vi "Afficheur.vi"() -> ()   [LabVIEW 2013]
uses:
  <vilib>/DAQmx/read.llb/DAQmx Read (Analog Wfm 1Chan NSamp).vi
  <vilib>/DAQmx/create/channels.llb/DAQmx Create Channel (AI-Voltage-Basic).vi
  <vilib>/DAQmx/configure/timing.llb/DAQmx Timing (Sample Clock).vi
  <vilib>/measure/matone.llb/Extract Single Tone Information 1 Chan.vi
  <vilib>/DAQmx/miscellaneous.llb/DAQmx Fill In Error Info.vi
  <vilib>/express/express analysis/Spectral/Block/exnSpectralBlock spectral measurements PSD poly.vi
  <vilib>/express/express analysis/Spectral/Block/exnSpectralBlock spectral measurements PSD WFM.vi
  <vilib>/express/express analysis/Spectral/XNode/ExpressSpectralMeasurementsBlockNode.xnode
  <vilib>/measure/NI_MAPro.lvlib
panel:
  in  "fenetre":dbl
  out "indice fractionnaire ou x":dbl
  out "Y":dbl[](array[numeric])
  out "Final Waveform":waveform(dbl)(graph)
  out "Valeur efficace":dbl
  out "?":cluster{"f0":dbl, "df":dbl, "magnitude":dbl[]}(graph)
  out "mean":dbl caption="moyenne" format="%0.2f"
  out "Fréquence":dbl
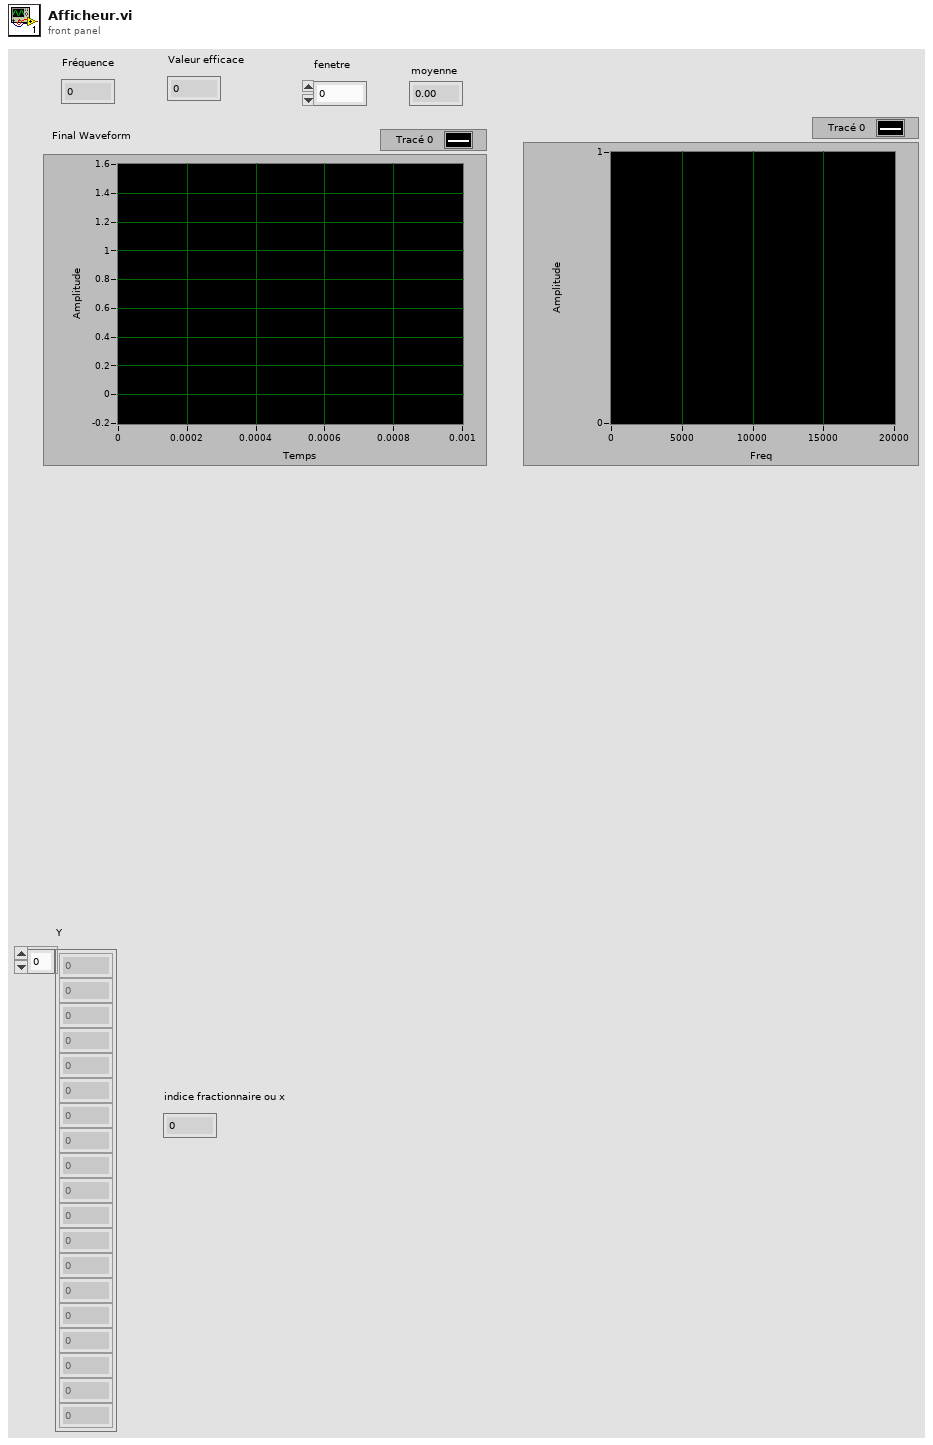
[diagram p1: front panel]
types:
  T1 = cluster{"averaging mode":u16, "weighting mode":u16, "number of averages":u32}
  T2 = cluster{"dB On (F)":bool, "unwrap phase (F)":bool, "convert to degree (F)":bool}
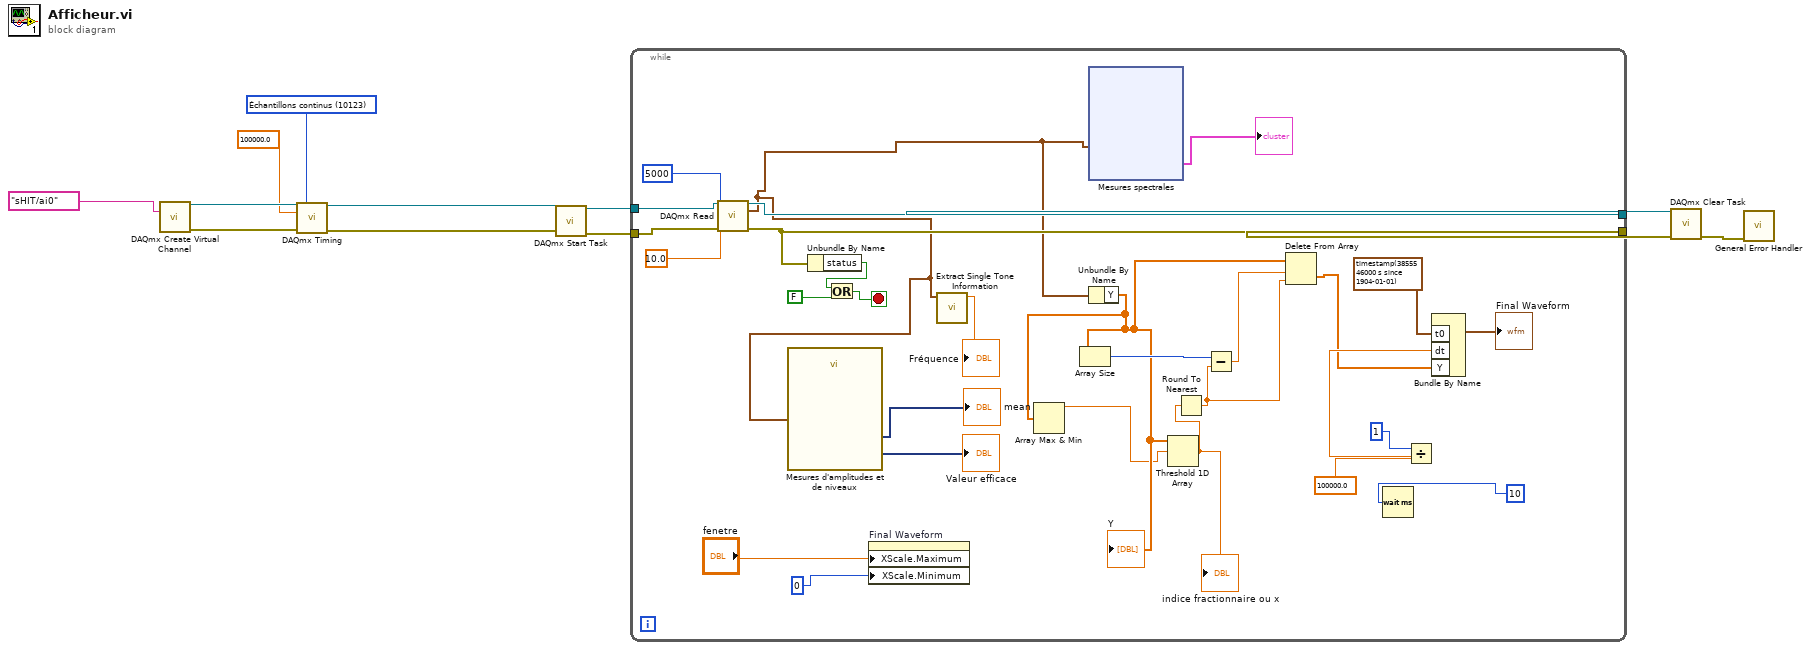
[diagram p0: block diagram]
diagram:
  w10 = 10123 items=["Échantillons finis"=10178, "Échantillons continus"=10123, "Point par point avec cadencement matériel"=12522] ("sample mode")
  n1 = call-poly <vilib>:"DAQmx Create Virtual Channel.vi"("physical channels"=tag "sHIT/ai0" ("Voie physique DAQmx")) -> ("task out"=w12:refnum<k21>, "error out"=w11:errorcluster)  [unwired: 13 in]
  n2 = call-poly <vilib>:"DAQmx Timing.vi"("task/channels in"=w12, "sample mode"=w10, "rate"=100000.0, "error in"=w11) -> ("task out"=w3:refnum<k21>, "error out"=w2:errorcluster)  [unwired: 10 in]
  n3 = call <vilib>:"DAQmx Start Task.vi"("task/channels in"=w3, "error in"=w2) -> ("task out"=w9:refnum<k21>, "error out"=w8:errorcluster)  [unwired: 12 in]
  n4 = while {
    tunnel: w9 -> [w41]
    tunnel: w8 -> [w40]
    tunnel: [w38] -> w7
    tunnel: [w34] -> w6
    stop <- w37 stop-if-true
    n5 = call-poly <vilib>:"DAQmx Read.vi"("task/channels in"=w41, "number of samples per channel"=5000, "timeout"=10.0, "error in"=w40) -> ("task out"=w38:refnum<k21>, "data"=w28:waveform(dbl), "error out"=w34:errorcluster)  [unwired: 9 in]
    n6 = call "Mesures d'amplitudes et de niveaux"("Signals"=w28) -> ("Mean (DC)"=→"mean":dynamicdata, "RMS"=→"Valeur efficace":dynamicdata)  [unwired: 12 in, 1 out]
    n7 = Unbundle By Name(w34) -> ("status"=w35:bool)
    n8 = Or(x=w35, y=FALSE) -> (x .or. y?=w37:bool)
    n9 = property on="Final Waveform" class="GraphWF (strict)"("XScale.Maximum"="fenetre", "XScale.Minimum"=0) -> ()  [unwired: 2 in, 2 out]
    n10 = call-poly <vilib>:"Extract Single Tone Information.vi"("time signal in"=w28) -> ("detected frequency"=→"Fréquence":dbl)  [unwired: 5 in, 5 out]
    n11 = xnode "Mesures spectrales"("Signaux"=w28) -> ("DSP"=→"?":cluster{"f0":dbl, "df":dbl, "magnitude":dbl[]})  [unwired: 1 in, 1 out]
    n12 = Unbundle By Name(w28) -> ("Y"=w17:dbl[])
    "Y" <- w17
    n13 = Array Max & Min(array=w17) -> (max value=w16:dbl)  [unwired: 3 out]
    n14 = Array Size(array=w17) -> (size(s)=w27:i32)
    n15 = Threshold 1D Array(2:w16, 3:w17) -> (0:w20:dbl)  [unwired: 1 in]
    "indice fractionnaire ou x" <- w20
    n16 = Round To Nearest(number=w20) -> (nearest integer value=w19:dbl)
    n17 = Subtract(x=w27, y=w19) -> (x-y=w18:dbl)
    n18 = Delete From Array(array=w17, length=w18, index=w19) -> (deleted portion=w15:dbl[])  [unwired: 1 out]
    n19 = Wait (ms)(milliseconds to wait=10) -> ()  [unwired: 1 out]
    n20 = Divide(x=1, y=100000.0) -> (x/y=w23:dbl)
    n21 = Bundle By Name("t0"=timestamp(3855546000 s since 1904-01-01), "dt"=w23, "Y"=w15) -> (→"Final Waveform":waveform(dbl))  [unwired: 1 in]
  }
  n22 = call <vilib>:"DAQmx Clear Task.vi"("task in"=w7, "error in"=w6) -> ("error out"=w5:errorcluster)  [unwired: 13 in]
  n23 = call <vilib>:"General Error Handler.vi"("error in (no error)"=w5) -> ()  [unwired: 10 in, 5 out]
